vi "Calculate Optimum Steer.vi"(5 "Rotation Only":bool, 7 "Previous Set Swerve":T1 {"Angle" scale format="%.3f"; "Velocity" scale=-1.0..1.0 scale format="%.1f"}, 11 "New Swerve":T1 {"Angle" scale format="%.3f"; "Velocity" scale=-1.0..1.0 scale format="%.1f"}) -> (3 "Set Swerve Out":T1 {"Angle" scale format="%.3f"; "Velocity" scale=-1.0..1.0 scale format="%.1f"})   [LabVIEW 2020, in "SwerveDrive_ACT_ts.lvlib"]
uses:
  SwerveDrive_ACT_ts.lvlib
  Shared Code/TypeDefs/Cluster_Module Velocity-Direction-Rotations.ctl
  Shared Code/TypeDefs/Level_Velocity plus-minus 1.ctl
  Shared Code/TypeDefs/Dial_Compase heading unit circle CCW positive.ctl
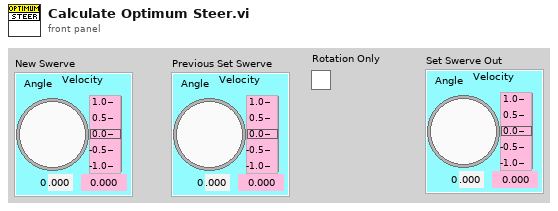
[diagram p1: front panel]
types:
  T1 = typedef "Cluster_Module Velocity-Direction-Rotations.ctl" = cluster{"Velocity":T2, "Angle":T3, "Rotations Count":dbl}
  T2 = typedef "Level_Velocity plus-minus 1.ctl" = dbl
  T3 = typedef "Dial_Compase heading unit circle CCW positive.ctl" = dbl
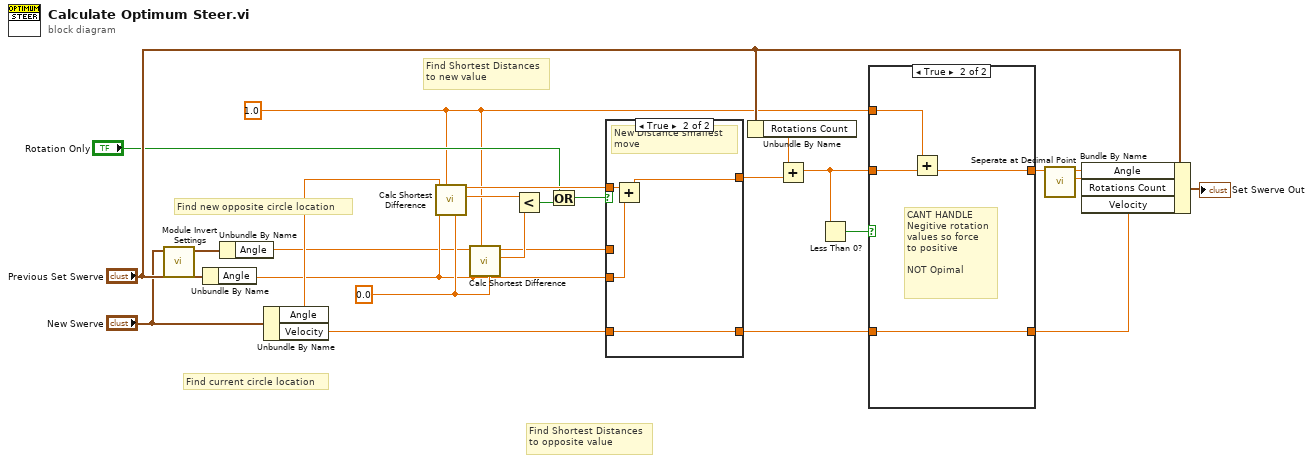
[diagram p0: block diagram]
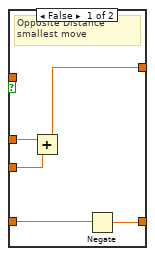
[diagram p3: hidden frame]
diagram:
  w21 = 0.0 ("Circle Min Value")
  w1 = 1.0 ("Circle Max Value")
  # "Find new opposite circle location"
  # "Find current circle location"
  # "Find Shortest Distances\nto opposite value"
  # "Find Shortest Distances\nto new value"
  n1 = call "Module Invert Settings.vi"("Setting"="New Swerve") -> ("Inverted Setting Out"=w11:T1)  [unwired: 10 in]
  n2 = Unbundle By Name("Previous Set Swerve") -> ("Angle"=w14:T3)
  n3 = Unbundle By Name(w11) -> ("Angle"=w10:T3)
  n4 = Unbundle By Name("New Swerve") -> ("Angle"=w19:T3, "Velocity"=w20:T2)
  n5 = call "Calc Shortest Difference.vi"("Min Value"=w21, "Max Value"=w1, "Previous Real Position"=w14, "New Real Position"=w19) -> ("Shortest Distance Out"=w26:dbl, "Shortest Direction Out"=w22:dbl)  [unwired: 6 in]
  n6 = call "Calc Shortest Difference.vi"("Min Value"=w21, "Max Value"=w1, "Previous Real Position"=w14, "New Real Position"=w10) -> ("Shortest Distance Out"=w25:dbl, "Shortest Direction Out"=w23:dbl)  [unwired: 6 in]
  n7 = Less?(x=w26, y=w25) -> (x < y?=w24:bool)
  n8 = Or(x="Rotation Only", y=w24) -> (x .or. y?=w8:bool)
  n9 = case shown="True" w8 {
    tunnel: [w31 w35] -> w13
    tunnel: w23 -> [w29 _]
    tunnel: w22 -> [_ w34]
    tunnel: w14 -> [w30 w33]
    tunnel: w20 -> [w28 w32]
    tunnel: [w27 w32] -> w3
    frame False {
      # "Opposite Distance smallest move"
      n10 = Add(x=w29, y=w30) -> (x+y=w31:T3)
      n11 = Negate(x=w28) -> (-x=w27:T2)
    }
    frame True {
      # "New Distance smallest move"
      n12 = Add(x=w34, y=w33) -> (x+y=w35:T3)
    }
  }
  n13 = Unbundle By Name("Previous Set Swerve") -> ("Rotations Count"=w17:dbl)
  n14 = Add(x=w17, y=w13) -> (x+y=w5:T3)
  n15 = Less Than 0?(x=w5) -> (x < 0?=w6:bool)
  n16 = case shown="True" w6 {
    tunnel: w5 -> [w37 w41]
    tunnel: [w37 w39] -> w4
    tunnel: w3 -> [w36 w38]
    tunnel: [w36 w38] -> w2
    tunnel: w1 -> [_ w40]
    frame False {
    }
    frame True {
      # "CANT HANDLE\nNegitive rotation\nvalues so force\nto positive\n\nNOT Opimal"
      n17 = Add(x=w40, y=w41) -> (x+y=w39:T3)
    }
  }
  n18 = call "Seperate at Decimal Point.vi"("Rotations"=w4) -> ("Rotations"=w16:dbl, "Angle"=w15:T3)  [unwired: 9 in]
  n19 = Bundle By Name(cluster="Previous Set Swerve", "Angle"=w15, "Rotations Count"=w16, "Velocity"=w2) -> (→"Set Swerve Out":T1)
